vi "SerRW-Array.vi"(0 "COMPORT":refnum<visa-resource-name>="COM4", 5 "Delay Time (ms)":dbl=1.0 caption="Delay Time (s)", 11 "error in (no error)":errorcluster, 12 "Command ( ; seperation)":string, 13 "Open Serial":bool, 14 "Close Serial":bool) -> (1 "time(s)":dbl=0.17611279999982798, 2 "Success":bool[](array[boolean]), 3 "All Success":bool, 4 "comport":refnum<visa-resource-name>="COM4", 6 "Array":string[](array[string]), 8 "string":string="caladc\r\n>\ncaladc -r\r\ncaladc delay: 0x00004333\r\n>\r\n", 15 "error out":errorcluster)   [LabVIEW 2018]
panel:
  out "output 2":string
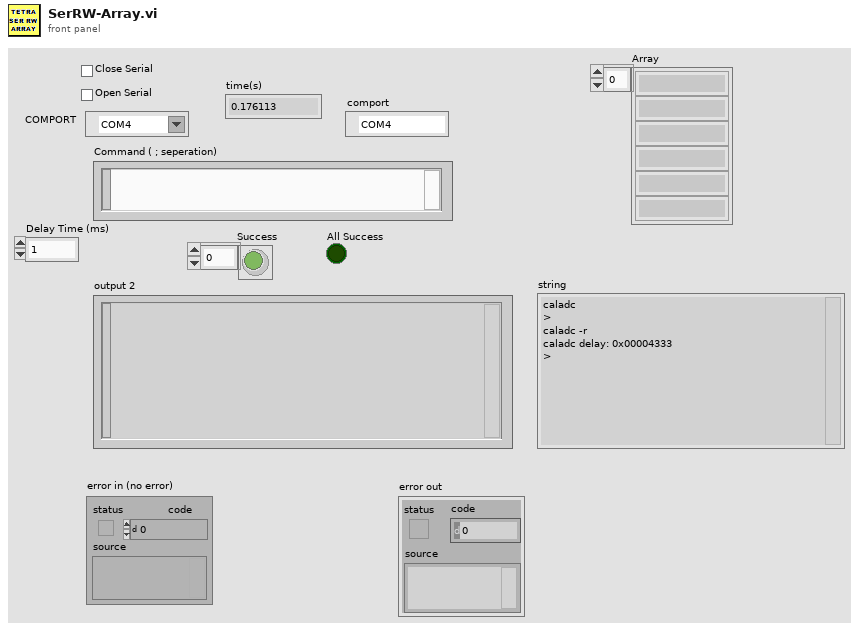
[diagram p1: front panel]
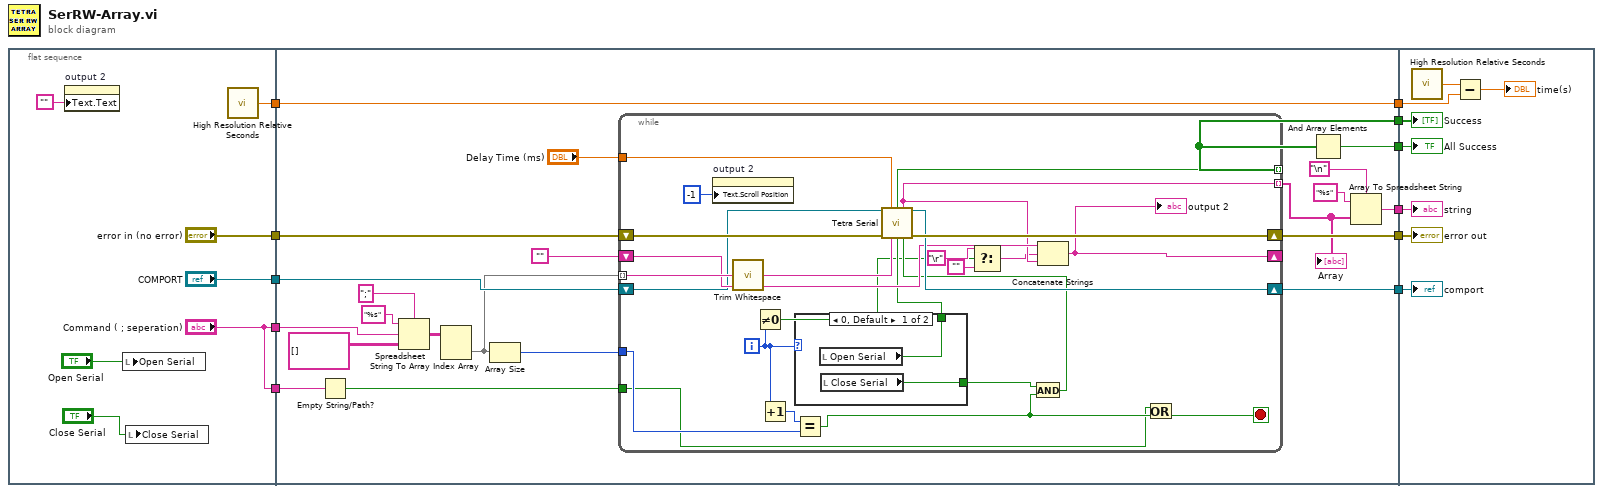
[diagram p0: block diagram]
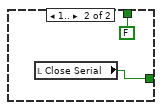
[diagram p2: hidden frame]
diagram:
  n1 = flat-sequence {
    tunnel: ["error in (no error)"] -> w6
    tunnel: ["COMPORT"] -> w5
    tunnel: ["Command ( ; seperation)"] -> w4
    tunnel: [w16] -> w3
    tunnel: ["Command ( ; seperation)"] -> w1
    tunnel: [w36] -> w11
    tunnel: [w33] -> w10
    tunnel: [w31] -> w9
    tunnel: [w26] -> w8
    tunnel: [w23] -> w7
    tunnel: w6 -> [w35]
    tunnel: w5 -> [w34]
    tunnel: w4 -> [w28]
    tunnel: w3 -> [w22]
    tunnel: [w22] -> w2
    tunnel: w1 -> [w20]
    tunnel: w11 -> [w74]
    tunnel: w10 -> [w75]
    tunnel: w9 -> [w76]
    tunnel: w8 -> [w77]
    tunnel: w7 -> [w73]
    tunnel: w2 -> [w71]
    frame #0 {
      n2 = property on="output 2" class="Str"("Text.Text"="") -> ()  [unwired: 2 in, 2 out]
      n3 = local write "Open Serial"("Open Serial") -> ()
      n4 = local write "Close Serial"("Close Serial") -> ()
      n5 = call <vilib>:"High Resolution Relative Seconds.vi"() -> ("relative seconds"=w16:dbl)
    }
    frame #1 {
      n6 = Empty String/Path?(string/path=w20) -> (empty?=w19:bool)
      n7 = Spreadsheet String To Array(delimiter (Tab)=";", format string="%s", spreadsheet string=w28, array type (2D Dbl)=string[][] []) -> (array=w37:string[][])
      n8 = Index Array(array=w37) -> (element=w32:string[])  [unwired: 2 in]
      n9 = Array Size(array=w32) -> (size(s)=w24:i32)
      n10 = while {
        shift-right: [w65] -> w36
        shift-left: w35 -> [w64]
        shift-right: [w63] -> w33
        shift-left: w34 -> [w55]
        tunnel: [w59] -> w25 mode=indexing
        tunnel: w32 -> [w62] mode=indexing
        tunnel: w24 -> [w52]
        shift-right: [w56] -> _
        shift-left: "" -> [w60]
        tunnel: [w57] -> w23 mode=indexing
        tunnel: "Delay Time (ms)" -> [w48]
        tunnel: w19 -> [w41]
        i -> [w44]
        stop <- w42 stop-if-true
        n11 = property on="output 2" class="Str"("Text.Scroll Position"=-1) -> ()  [unwired: 2 in, 2 out]
        n12 = call <vilib>:"Trim Whitespace.vi"("string"=w62) -> ("trimmed string"=w58:string)  [unwired: 1 in]
        n13 = Not Equal To 0?(x=w44) -> (x != 0?=w45:bool)
        n14 = Increment(x=w44) -> (x+1=w53:i32)
        n15 = case shown="0, Default" w44 {
          tunnel: [w67 FALSE ("Open Serial")] -> w54
          tunnel: [w66 w68] -> w50
          frame 0, Default {
            n16 = local read "Open Serial"() -> (w67:bool)
            n17 = local read "Close Serial"() -> (w66:bool)
          }
          frame 1.. {
            n18 = local read "Close Serial"() -> (w68:bool)
          }
        }
        n19 = Equal?(x=w53, y=w52) -> (x = y?=w51:bool)
        n20 = Select(t="\r", s=w45, f="") -> (s? t:f=w47:string)
        n21 = And(x=w50, y=w51) -> (x .and. y?=w49:bool)
        n22 = call "Tetra Serial.vi"("COMPORT"=w55, "Delay Time (ms)"=w48, "error in (no error)"=w64, "Command"=w58, "Open Ser(t)"=w54, "Close Ser(t)"=w49) -> ("Success"=w57:bool, "output"=w59:string, "comport"=w63:refnum<visa-resource-name>, "error out"=w65:errorcluster)  [unwired: 5 in, 1 out]
        n23 = Concatenate Strings(w60, w47, w59) -> (w56:string)
        "output 2" <- w56
        n24 = Or(x=w41, y=w51) -> (x .or. y?=w42:bool)
      }
      "Array" <- w25
      n25 = And Array Elements(Boolean array=w23) -> (logical AND=w26:bool)
      n26 = Array To Spreadsheet String(delimiter (Tab)="\n", array=w25, 3:"%s" ("format string")) -> (spreadsheet string=w31:string)
    }
    frame #2 {
      n27 = call <vilib>:"High Resolution Relative Seconds.vi"() -> ("relative seconds"=w72:dbl)
      n28 = Subtract(x=w72, y=w71) -> (x-y=→"time(s)":dbl)
      "error out" <- w74
      "comport" <- w75
      "Success" <- w73
      "string" <- w76
      "All Success" <- w77
    }
  }
